vi "Close.vi"(8 "error in":errorcluster, 11 "MSS in":refnum<class "Measure and Stimulus Subsystems.lvclass">) -> (0 "error out":errorcluster, 3 "MSS out":refnum<class "Measure and Stimulus Subsystems.lvclass">)   [LabVIEW 2023, in "HAL GOOP4.lvlib" / "Measure and Stimulus Subsystems.lvclass"]
uses:
  Measure and Stimulus Subsystems.lvclass
  Measure and Stimulus Subsystems.lvclass/Measure and Stimulus Subsystems.ctl
  Instrument/utils/Instrument_GetAttributes.vi
  Interfaces/IConfigure/IConfigure.lvclass
  Instrument/Instrument.lvclass
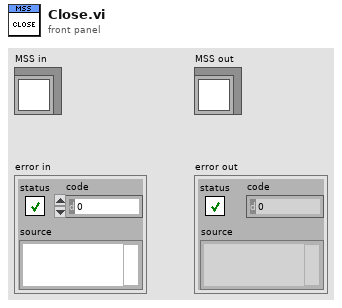
[diagram p1: front panel]
types:
  T1 = map{string, cluster{"Instrument":refnum<class "Instrument.lvclass">, "Ref Count":u8}}
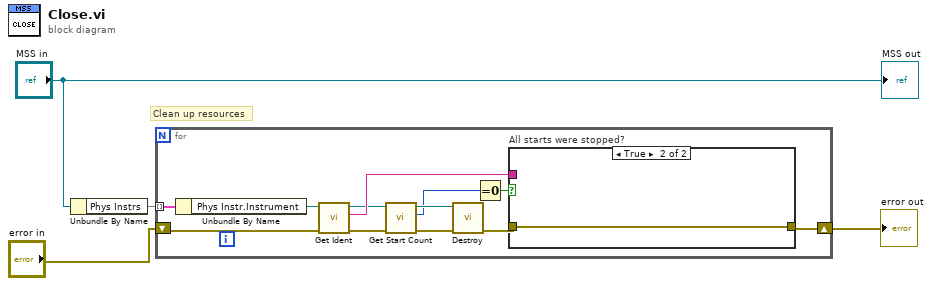
[diagram p0: block diagram]
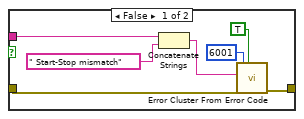
[diagram p2: hidden frame]
diagram:
  # "Clean up resources"
  n1 = Unbundle By Name("MSS in") -> ("Phys Instrs"=w4:T1)
  n2 = for {
    tunnel: w4 -> [w16] mode=indexing
    shift-right: [w13] -> w2
    shift-left: "error in" -> [w15]
    n3 = Unbundle By Name(w16) -> ("Phys Instr.Instrument"=w10:refnum<class "Instrument.lvclass">)
    n4 = call "Get Ident.vi"("Error In"=w15, "reference in"=w10) -> ("Error Out"=w11:errorcluster, "Instr Ident"=w9:string, "reference out"=w7:refnum<class "Instrument.lvclass">)  [unwired: 7 in]
    n5 = call "Get Start Count.vi"("Error In"=w11, "reference in"=w7) -> ("Error Out"=w8:errorcluster, "Start Count"=w5:i16, "reference out"=w6:refnum<class "Instrument.lvclass">)  [unwired: 7 in]
    n6 = call "Destroy.vi"("Error In"=w8, "reference in"=w6) -> ("Error Out"=w14:errorcluster)  [unwired: 8 in, 1 out]
    n7 = Equal To 0?(x=w5) -> (x = 0?=w12:bool)
    n8 = case "All starts were stopped?" shown="True" w12 {
      tunnel: w14 -> [w23 w24]
      tunnel: [w22 w24] -> w13
      tunnel: w9 -> [w20 _]
      frame False {
        n9 = Concatenate Strings(w20, " Start-Stop mismatch" ("string")) -> (w18:string)
        n10 = call <vilib>:"Error Cluster From Error Code.vi"("show call chain? (False)"=TRUE, "error in (no error)"=w23, "error message (\"\")"=w18, "error code (0)"=6001) -> ("error out"=w22:errorcluster)  [unwired: 5 in]
      }
      frame True {
      }
    }
  }
  "error out" <- w2
  "MSS out" <- "MSS in"
